vi "Stepper Motor 2.3 Working.vi"(9 "Dir":bool=TRUE, 10 "y (inches)":dbl) -> ()   [LabVIEW 2017]
uses:
  <vilib>/myRIO/Instrument Drivers/Onboard IO/DIO/typedefs/DIO Reference.ctl
  <vilib>/myRIO/Common/Instrument Driver Framework/Utilities/typedefs/myRIO Generic Hardware Reference.ctl
  <vilib>/myRIO/Common/Instrument Driver Framework/Utilities/typedefs/Hardware Version Enum.ctl
  <vilib>/myRIO/Common/Instrument Driver Framework/Utilities/typedefs/myRIO v1.0 Reference.ctl
  <vilib>/myRIO/Common/Instrument Driver Framework/Utilities/typedefs/Generic FPGA Reference.ctl
  <vilib>/myRIO/Common/Instrument Driver Framework/myRIO v1.0/DIO/typedefs/DIO Channels List.ctl
  <vilib>/myRIO/Common/Instrument Driver Framework/myRIO v1.0/DIO/typedefs/DIO Channels Enum.ctl
  <vilib>/userdefined/High Color/nirio_resource_hc.ctl
  <vilib>/myRIO/Common/Instrument Driver Framework/Utilities/vis/Is FPGA Ref Available.vi
  <vilib>/myRIO/Common/Instrument Driver Framework/myRIO v1.0/DIO/vis/myRIO v1.1 Open DIO.vi
  <vilib>/myRIO/Instrument Drivers/Onboard IO/DIO/vis/Write.vi
  <vilib>/myRIO/Instrument Drivers/Onboard IO/DIO/vis/Read.vi
  <vilib>/myRIO/Common/Instrument Driver Framework/Utilities/vis/Validate Channels.vi
  <vilib>/myRIO/Common/Instrument Driver Framework/myRIO v1.0/DIO/vis/myRIO v1.0 Reserve DIO.vi
  <vilib>/myRIO/Common/Instrument Driver Framework/myRIO v1.0/Resource Manager/vis/myRIO v1.0 Reserve Channel List.vi
  <vilib>/myRIO/Common/Instrument Driver Framework/myRIO v1.0/DIO/vis/myRIO v1.0 Build MUX Configuration DIO.vi
  <vilib>/myRIO/Common/Instrument Driver Framework/myRIO v1.0/Resource Manager/vis/myRIO v1.0 Reserve Channel.vi
  <vilib>/myRIO/Common/Instrument Driver Framework/myRIO v1.0/Resource Manager/vis/myRIO v1.0 Unreserve Channel.vi
  <vilib>/myRIO/Common/Instrument Driver Framework/myRIO v1.0/Resource Manager/vis/myRIO v1.0 Create Configuration List.vi
  <vilib>/myRIO/Common/Instrument Driver Framework/myRIO v1.0/Resource Manager/vis/myRIO v1.0 Build Mutex Name.vi
  <vilib>/Utility/VariantDataType/GetNumericInfo.vi
  <vilib>/Utility/error.llb/Error Cluster From Error Code.vi
  <vilib>/myRIO/Common/Instrument Driver Framework/myRIO v1.0/myRIO v1.1 Open.vi
  <vilib>/myRIO/Common/Instrument Driver Framework/Utilities/vis/IO Manager.vi
  <vilib>/myRIO/Common/Instrument Driver Framework/Utilities/vis/Configuration Manager.vi
  <vilib>/myRIO/Common/Instrument Driver Framework/myRIO v1.0/Resource Manager/vis/myRIO v1.0 Configure IO.vi
  <vilib>/myRIO/Common/Instrument Driver Framework/myRIO v1.0/myRIO v1.0 Close.vi
  <vilib>/myRIO/Common/Instrument Driver Framework/myRIO v1.0/DIO/vis/myRIO v1.0 Write DIO.vi
  <vilib>/myRIO/Common/Instrument Driver Framework/myRIO v1.0/DIO/vis/myRIO v1.0 Read DIO.vi
  <vilib>/myRIO/Express VI/Onboard Devices/LED/LED Express VI.xnode
  <vilib>/myRIO/Instrument Drivers/Onboard IO/DIO/vis/myRIO DIO Open.xnode
  <vilib>/myRIO/Express VI/Onboard IO/DO/DO Express VI.xnode
  <vilib>/myRIO/Express VI/Onboard IO/DI/DI Express VI.xnode
  <vilib>/myRIO/Instrument Drivers/Onboard IO/DIO/DIO.lvlib
panel:
  out "current pps d":dbl
  out "loop num d":i32
  out "nc":dbl format="%.2f"
  out "current pps c":dbl
  out "loop num c":i32
  out "na":dbl format="%.2f"
  out "current pps a":dbl
  out "loop num a":i32
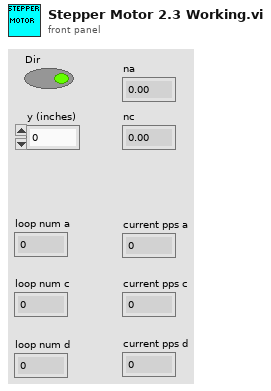
[diagram p1: front panel]
types:
  T1 = typedef "DIO.lvlib/DIO Reference.ctl" = cluster{"myRIO Reference":T2, "DIO Channels List":T6}
  T2 = typedef "myRIO Generic Hardware Reference.ctl" = cluster{"myRIO Model":T3, "myRIO Hardware Reference":T4}
  T3 = typedef "Hardware Version Enum.ctl" = enum16{"Unknown", "myRIO-1900", "myRIO-1950", "roboRIO", "NI ELVIS RIO CM"}
  T4 = typedef "myRIO v1.0 Reference.ctl" = cluster{"Generic FPGA Reference":T5, "Allow multiple opens":bool}
  T5 = typedef "Generic FPGA Reference.ctl" = refnum<k20>
  T6 = typedef "DIO Channels List.ctl" = T7[]
  T7 = typedef "DIO Channels Enum.ctl" = enum16{"Not Connected", "C/DIO0", "C/DIO1", "C/DIO2", "C/DIO3", "C/DIO4", "C/DIO5", "C/DIO6", "C/DIO7", "A/DIO0", "A/DIO1", "A/DIO2", "A/DIO3", "A/DIO4", "A/DIO5", "A/DIO6", "A/DIO7", "A/DIO8", "A/DIO9", "A/DIO10", "A/DIO11", "A/DIO12", "A/DIO13", "A/DIO14", "A/DIO15", "B/DIO0", "B/DIO1", "B/DIO2", "B/DIO3", "B/DIO4", "B/DIO5", "B/DIO6", "B/DIO7", "B/DIO8", "B/DIO9", "B/DIO10", "B/DIO11", "B/DIO12", "B/DIO13", "B/DIO14", "B/DIO15", "LED0", "LED1", "LED2", "LED3", "Button0", "DIO/DIO0", "DIO/DIO1", "DIO/DIO2", "DIO/DIO3", "DIO/DIO4", "DIO/DIO5", "DIO/DIO6", "DIO/DIO7", "DIO/DIO8", "DIO/DIO9", "SPI/CS0", "SPI/CS1", "SPI/CS2", "SPI/CS3", "LED RADIO (Green)", "LED RADIO (Red)", "LED COMM (Green)", "LED COMM (Red)", "LED MODE (Green)", "LED MODE (Red)"}
  T8 = typedef "nirio_resource_hc.ctl" = tag
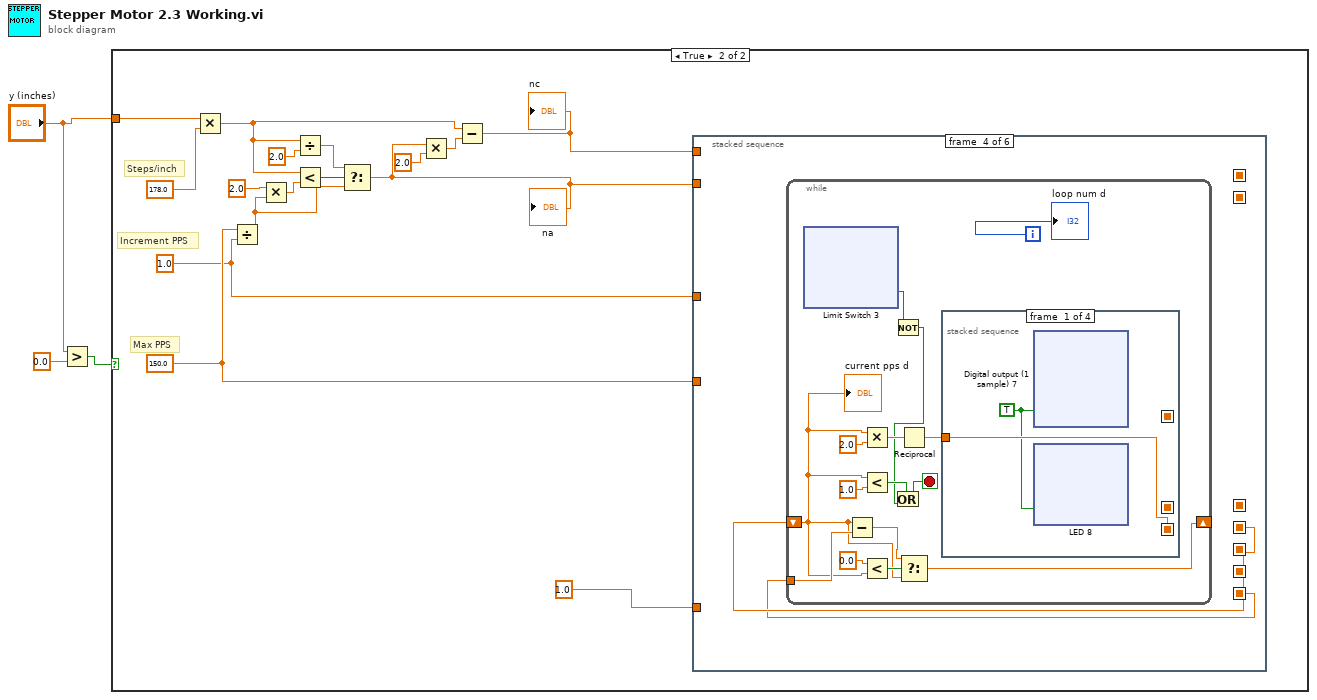
[diagram p0: block diagram]
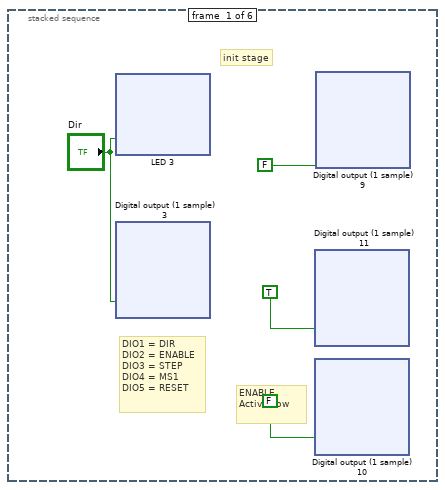
[diagram p3: hidden frame]
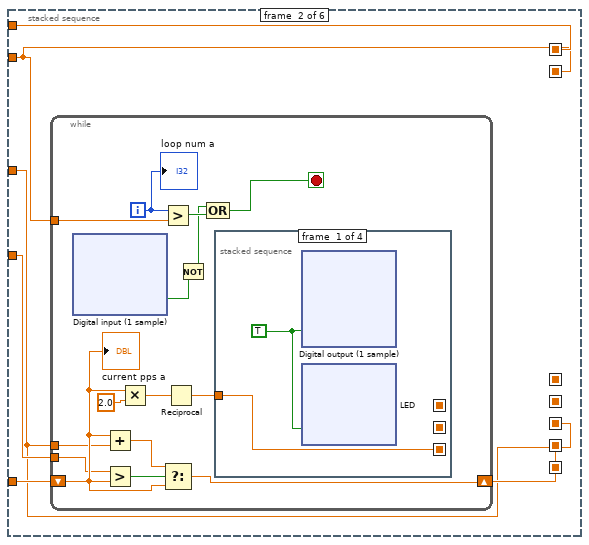
[diagram p4: hidden frame]
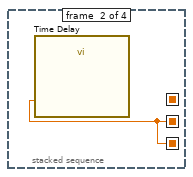
[diagram p5: hidden frame]
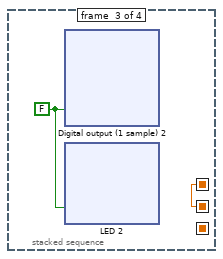
[diagram p6: hidden frame]
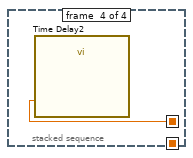
[diagram p7: hidden frame]
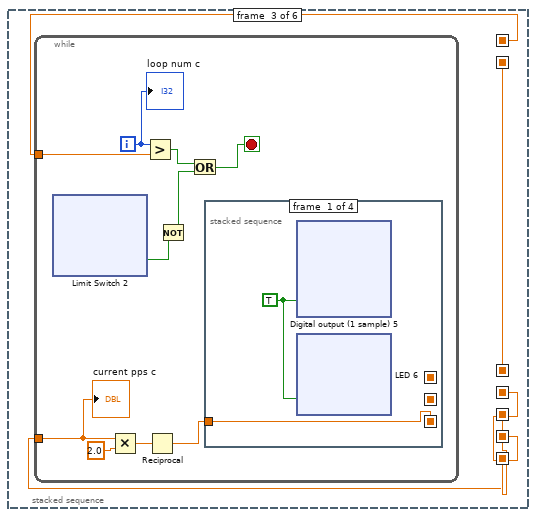
[diagram p8: hidden frame]
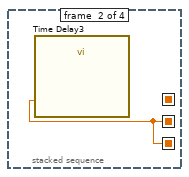
[diagram p9: hidden frame]
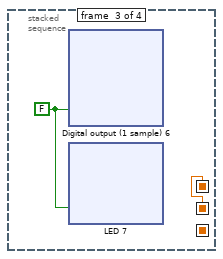
[diagram p10: hidden frame]
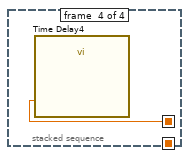
[diagram p11: hidden frame]
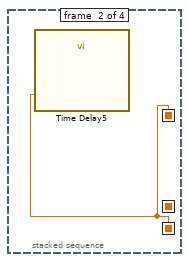
[diagram p12: hidden frame]
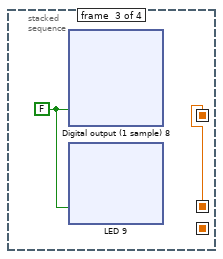
[diagram p13: hidden frame]
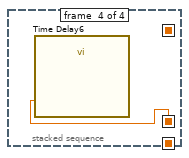
[diagram p14: hidden frame]
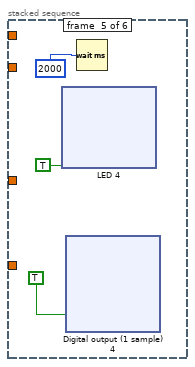
[diagram p15: hidden frame]
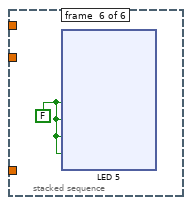
[diagram p16: hidden frame]
diagram:
  n1 = Greater?(x="y (inches)", y=0.0) -> (0:w1:bool)
  n2 = case shown="True" w1 {
    tunnel: "y (inches)" -> [_ w18]
    frame False {
    }
    frame True {
      w15 = 1.0 ("increment pps")
      w16 = 150.0 ("max pps")
      # "Increment PPS"
      # "Steps/inch"
      # "Max PPS"
      n3 = Multiply(x=w18, y=178.0 ("steps/in")) -> (x*y=w7:dbl)
      n4 = Divide(x=w16, y=w15) -> (x/y=w4:dbl)
      n5 = Multiply(x=2.0 ("y"), y=w4) -> (x*y=w14:dbl)
      n6 = Divide(x=w7, y=2.0) -> (x/y=w11:dbl)
      n7 = Less?(x=w7, y=w14) -> (x < y?=w13:bool)
      n8 = Select(t=w11, s=w13, f=w4) -> (s? t:f=w8:dbl)
      "na" <- w8
      n9 = Multiply(x=w8, y=2.0) -> (x*y=w10:dbl)
      n10 = Subtract(x=w7, y=w10) -> (x-y=w6:dbl)
      "nc" <- w6
      n11 = stacked-sequence {
        seq-local: [_ w202 _ _ _ _] -> [_ _ w401 _ _ _]
        seq-local: [_ w201 _ _ _ _] -> [_ _ w402 _ _ _]
        seq-local: [_ w200 _ _ _ _] -> [_ _ w404 _ _ _]
        seq-local: [_ w199 _ _ _ _] -> [_ _ w403 _ _ _]
        seq-local: [_ _ w404 _ _ _] -> [_ _ _ w596 _ _]
        seq-local: [_ _ w403 _ _ _] -> [_ _ _ _ _ _]
        seq-local: [_ _ w402 _ _ _] -> [_ _ _ w597 _ _]
        tunnel: w16 -> [_ w204 _ _ _ _]
        tunnel: w15 -> [_ w200 _ _ _ _]
        tunnel: 1.0 ("starting pps") -> [_ w203 _ _ _ _]
        tunnel: w8 -> [_ w199 _ _ _ _]
        tunnel: w6 -> [_ w202 _ _ _ _]
        frame #0 {
          # "init stage"
          # "ENABLE\nActive Low"
          # "DIO1 = DIR\nDIO2 = ENABLE\nDIO3 = STEP\nDIO4 = MS1\nDIO5 = RESET"
          n12 = xnode "LED 3"("LED0"="Dir") -> ()  [unwired: 1 in, 1 out]
          n13 = xnode "Digital output (1 sample) 3"("DIR (A/DIO1 (Pin 13))"="Dir") -> ()  [unwired: 1 in, 1 out]
          n14 = xnode "Digital output (1 sample) 11"("A/DIO5 (Pin 21)"=TRUE) -> ()  [unwired: 1 in, 1 out]
          n15 = xnode "Digital output (1 sample) 10"("A/DIO2 (Pin 15)"=FALSE) -> ()  [unwired: 1 in, 1 out]
          n16 = xnode "Digital output (1 sample) 9"("A/DIO4 (Pin 19)"=FALSE) -> ()  [unwired: 1 in, 1 out]
        }
        frame #1 {
          n17 = while {
            shift-right: [w214] -> w201
            shift-left: w203 -> [w213]
            tunnel: w204 -> [w212]
            tunnel: w200 -> [w211]
            tunnel: w199 -> [w210]
            i -> [w209]
            stop <- w206 stop-if-true
            n18 = xnode "Digital input (1 sample)"() -> ("A/DIO0 (Pin 11)"=w207:bool)  [unwired: 1 in, 1 out]
            n19 = Add(x=w213, y=w211) -> (x+y=w215:dbl)
            n20 = Greater?(x=w212, y=w213) -> (0:w216:bool)
            n21 = Multiply(x=w213, y=2.0) -> (x*y=w219:dbl)
            n22 = Greater?(x=w209, y=w210) -> (0:w208:bool)
            n23 = Select(t=w215, s=w216, f=w213) -> (s? t:f=w214:dbl)
            n24 = Reciprocal(x=w219) -> (1/x=w217:dbl)
            n25 = Not(x=w207) -> (.not. x?=w205:bool)
            n26 = Compound Arithmetic op=OR(w205, w208) -> (w206:bool)
            n27 = stacked-sequence {
              seq-local: [w256 _ _ _] -> [_ w327 _ _]
              seq-local: [_ w327 _ _] -> [_ _ w329 _]
              seq-local: [_ _ w329 _] -> [_ _ _ w400]
              tunnel: w217 -> [w256 _ _ _]
              frame #0 {
                w255 = TRUE
                n28 = xnode "Digital output (1 sample)"("A/DIO3 (Pin 17)"=w255) -> ()  [unwired: 1 in, 1 out]
                n29 = xnode "LED"("LED1"=w255) -> ()  [unwired: 1 in, 1 out]
              }
              frame #1 {
                n30 = call "Time Delay"("Delay Time (s)"=w327) -> ()  [unwired: 10 in, 1 out]
              }
              frame #2 {
                w328 = FALSE
                n31 = xnode "Digital output (1 sample) 2"("A/DIO3 (Pin 17)"=w328) -> ()  [unwired: 1 in, 1 out]
                n32 = xnode "LED 2"("LED1"=w328) -> ()  [unwired: 1 in, 1 out]
              }
              frame #3 {
                n33 = call "Time Delay2"("Delay Time (s)"=w400) -> ()  [unwired: 10 in, 1 out]
              }
            }
            "current pps a" <- w213
            "loop num a" <- w209
          }
        }
        frame #2 {
          n34 = while {
            tunnel: w401 -> [w410]
            tunnel: w402 -> [w411]
            i -> [w409]
            stop <- w405 stop-if-true
            n35 = xnode "Limit Switch 2"() -> ("A/DIO0 (Pin 11)"=w408:bool)  [unwired: 1 in, 1 out]
            n36 = Multiply(x=w411, y=2.0) -> (x*y=w414:dbl)
            n37 = Greater?(x=w409, y=w410) -> (0:w406:bool)
            n38 = Reciprocal(x=w414) -> (1/x=w412:dbl)
            n39 = Not(x=w408) -> (.not. x?=w407:bool)
            n40 = Or(x=w406, y=w407) -> (x .or. y?=w405:bool)
            n41 = stacked-sequence {
              seq-local: [w451 _ _ _] -> [_ w522 _ _]
              seq-local: [_ w522 _ _] -> [_ _ w524 _]
              seq-local: [_ _ w524 _] -> [_ _ _ w595]
              tunnel: w412 -> [w451 _ _ _]
              frame #0 {
                w450 = TRUE
                n42 = xnode "Digital output (1 sample) 5"("A/DIO3 (Pin 17)"=w450) -> ()  [unwired: 1 in, 1 out]
                n43 = xnode "LED 6"("LED1"=w450) -> ()  [unwired: 1 in, 1 out]
              }
              frame #1 {
                n44 = call "Time Delay3"("Delay Time (s)"=w522) -> ()  [unwired: 10 in, 1 out]
              }
              frame #2 {
                w523 = FALSE
                n45 = xnode "Digital output (1 sample) 6"("A/DIO3 (Pin 17)"=w523) -> ()  [unwired: 1 in, 1 out]
                n46 = xnode "LED 7"("LED1"=w523) -> ()  [unwired: 1 in, 1 out]
              }
              frame #3 {
                n47 = call "Time Delay4"("Delay Time (s)"=w595) -> ()  [unwired: 10 in, 1 out]
              }
            }
            "current pps c" <- w411
            "loop num c" <- w409
          }
        }
        frame #3 {
          n48 = while {
            shift-right: [w604] -> _
            shift-left: w597 -> [w602]
            tunnel: w596 -> [w606]
            i -> [w603]
            stop <- w600 stop-if-true
            n49 = xnode "Limit Switch 3"() -> ("A/DIO0 (Pin 11)"=w599:bool)  [unwired: 1 in, 1 out]
            n50 = Subtract(x=w602, y=w606) -> (x-y=w608:dbl)
            n51 = Multiply(x=w602, y=2.0) -> (x*y=w611:dbl)
            n52 = Less?(x=w602, y=1.0) -> (x < y?=w612:bool)
            n53 = Less?(x=0.0, y=w602) -> (x < y?=w609:bool)
            n54 = Not(x=w599) -> (.not. x?=w598:bool)
            n55 = Or(x=w612, y=w598) -> (x .or. y?=w600:bool)
            n56 = Reciprocal(x=w611) -> (1/x=w607:dbl)
            n57 = Select(t=w608, s=w609, f=w602) -> (s? t:f=w604:dbl)
            n58 = stacked-sequence {
              seq-local: [w649 _ _ _] -> [_ w720 _ _]
              seq-local: [_ w720 _ _] -> [_ _ w722 _]
              seq-local: [_ _ w722 _] -> [_ _ _ w793]
              tunnel: w607 -> [w649 _ _ _]
              frame #0 {
                w648 = TRUE
                n59 = xnode "Digital output (1 sample) 7"("A/DIO3 (Pin 17)"=w648) -> ()  [unwired: 1 in, 1 out]
                n60 = xnode "LED 8"("LED1"=w648) -> ()  [unwired: 1 in, 1 out]
              }
              frame #1 {
                n61 = call "Time Delay5"("Delay Time (s)"=w720) -> ()  [unwired: 10 in, 1 out]
              }
              frame #2 {
                w721 = FALSE
                n62 = xnode "Digital output (1 sample) 8"("A/DIO3 (Pin 17)"=w721) -> ()  [unwired: 1 in, 1 out]
                n63 = xnode "LED 9"("LED1"=w721) -> ()  [unwired: 1 in, 1 out]
              }
              frame #3 {
                n64 = call "Time Delay6"("Delay Time (s)"=w793) -> ()  [unwired: 10 in, 1 out]
              }
            }
            "loop num d" <- w603
            "current pps d" <- w602
          }
        }
        frame #4 {
          n65 = xnode "LED 4"("LED2"=TRUE) -> ()  [unwired: 1 in, 1 out]
          n66 = xnode "Digital output (1 sample) 4"("A/DIO2 (Pin 15)"=TRUE) -> ()  [unwired: 1 in, 1 out]
          n67 = Wait (ms)(milliseconds to wait=u32 2000) -> ()  [unwired: 1 out]
        }
        frame #5 {
          w867 = FALSE
          n68 = xnode "LED 5"("LED0"=w867, "LED1"=w867, "LED2"=w867, "LED3"=w867) -> ()  [unwired: 1 in, 1 out]
        }
      }
    }
  }
